vi "GetHistoTdmConfig.vi"(0 "storage refnum (file) out":refnum<k20>, 1 "error in":errorcluster) -> (2 "storage refnum (file) out 2":refnum<k20>, 3 "output cluster":T1={"AutoLevel"=FALSE, "Thresold"=1.0, "Impedance "=1000000.0, "Voltage Range"=5.0, "Active Edge "=1} {"Active Edge" items=["Positive", "Negative"]; "Impedance" items=["50"=50.0, "1E+6"=1000000.0]}, 4 "error out":errorcluster)   [LabVIEW 2014]
uses:
  Configs/Count/Channel.ctl
  <vilib>/Platform/storage/lvStorage.llb/_queryPropPoly.vi
  <vilib>/Platform/storage/lvStorage.llb/_queryPropString.vi
  <vilib>/Platform/storage/lvStorage.llb/_queryGenericObjects.vi
  <vilib>/Platform/storage/lvStorage.llb/_loadAllDdt.vi
  <vilib>/Platform/storage/lvStorage.llb/xStorage/xStorageSupp/ErrorOut.vi
  <vilib>/Platform/storage/lvStorage.llb/xStorage/Read Data/Read Data.xnode
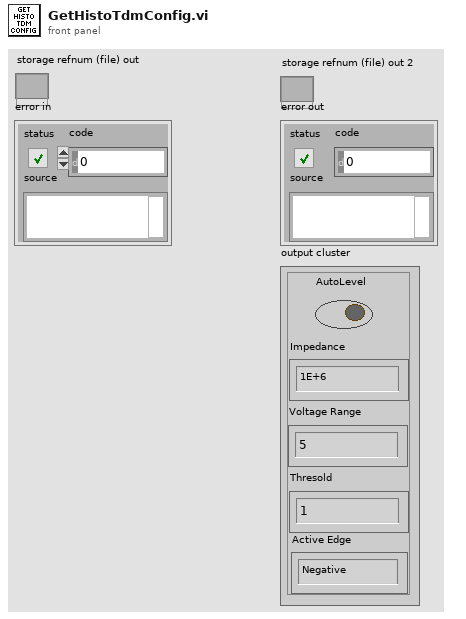
[diagram p1: front panel]
types:
  T1 = typedef "Channel.ctl" = cluster{"AutoLevel":bool, "Thresold":dbl, "Impedance ":dbl, "Voltage Range":dbl, "Active Edge ":i32}
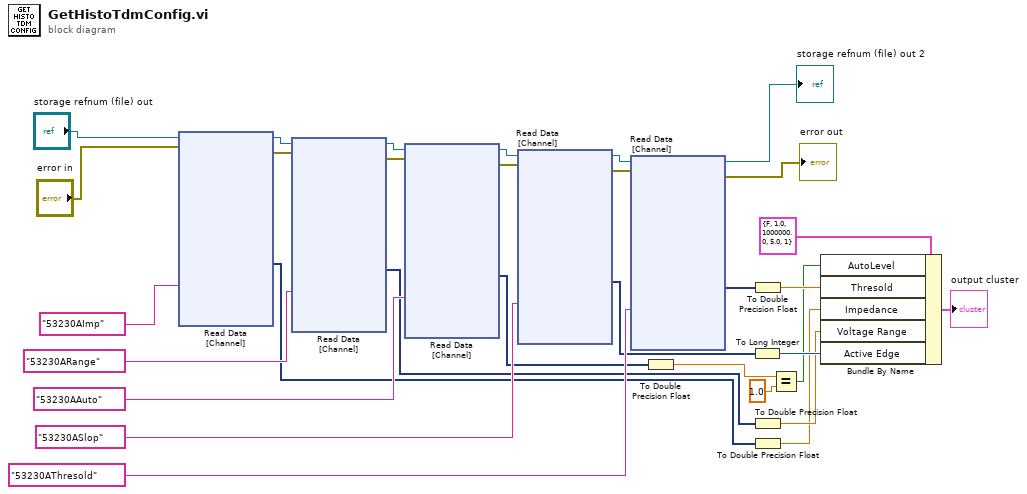
[diagram p0: block diagram]
diagram:
  n1 = xnode "Read Data\n[Channel]"("Name"="53230AImp", "storage refnum (file)"="storage refnum (file) out", "error in"="error in") -> ("Signal"=w7:dynamicdata, "storage refnum (file) out"=w31:refnum<k20>, "error out"=w30:errorcluster)  [unwired: 3 in, 1 out]
  n2 = xnode "Read Data\n[Channel]"("Name"="53230ARange", "storage refnum (file)"=w31, "error in"=w30) -> ("Signal"=w9:dynamicdata, "storage refnum (file) out"=w29:refnum<k20>, "error out"=w28:errorcluster)  [unwired: 3 in, 1 out]
  n3 = xnode "Read Data\n[Channel]"("Name"="53230AAuto", "storage refnum (file)"=w29, "error in"=w28) -> ("Signal"=w11:dynamicdata, "storage refnum (file) out"=w27:refnum<k20>, "error out"=w26:errorcluster)  [unwired: 3 in, 1 out]
  n4 = xnode "Read Data\n[Channel]"("Name"="53230ASlop", "storage refnum (file)"=w27, "error in"=w26) -> ("Signal"=w15:dynamicdata, "storage refnum (file) out"=w21:refnum<k20>, "error out"=w20:errorcluster)  [unwired: 3 in, 1 out]
  n5 = xnode "Read Data\n[Channel]"("Name"="53230AThresold", "storage refnum (file)"=w21, "error in"=w20) -> ("Signal"=w17:dynamicdata, "storage refnum (file) out"=→"storage refnum (file) out 2":refnum<k20>, "error out"=→"error out":errorcluster)  [unwired: 3 in, 1 out]
  n6 = To Double Precision Float(number=w11) -> (double precision float=w12:dbl)
  n7 = To Long Integer(number=w15) -> (32bit integer=w14:i32)
  n8 = To Double Precision Float(number=w17) -> (double precision float=w16:dbl)
  n9 = To Double Precision Float(number=w9) -> (double precision float=w8:dbl)
  n10 = To Double Precision Float(number=w7) -> (double precision float=w6:dbl)
  n11 = Equal?(x=w12, y=1.0) -> (x = y?=w10:bool)
  n12 = Bundle By Name(cluster=T1 {"AutoLevel"=FALSE, "Thresold"=1.0, "Impedance "=1000000.0, "Voltage Range"=5.0, "Active Edge "=1} ("Channel1"), "AutoLevel"=w10, "Thresold"=w16, "Impedance"=w6, "Voltage Range"=w8, "Active Edge"=w14) -> (→"output cluster":T1)
